vi "Measure.vi"(8 "error in (no error)":errorcluster, 11 "Measurement in":refnum<class "Measurement.lvclass">) -> (0 "error out":errorcluster, 3 "Measurement out":refnum<class "Measurement.lvclass">)   [LabVIEW 2016, in "Measurement Actor.lvlib" / "Measurement.lvclass"]
uses:
  Measurement.lvclass
  C:/Program Files (x86)/National Instruments/LabVIEW 2016/vi.lib/ActorFramework/Actor/Actor.lvclass
  Measurement.lvclass/Measurement.ctl
  <vilib>/ActorFramework/Actor/Actor.lvclass/Actor.ctl
  <vilib>/ActorFramework/Message Enqueuer/Message Enqueuer.lvclass/Message Enqueuer.ctl
  <vilib>/ActorFramework/Message Enqueuer/Init from Existing Queue.vi
  <vilib>/ActorFramework/Message Enqueuer/Enqueue.vi
  Messages/Acquire Msg/Acquire Msg.lvclass
  C:/Program Files (x86)/National Instruments/LabVIEW 2016/vi.lib/ActorFramework/Message/Message.lvclass
  Messages/Close Msg/Close Msg.lvclass
  <vilib>/ActorFramework/Message Priority Queue/Priority Enqueue.vi
  <vilib>/ActorFramework/Message Enqueuer/Message Enqueuer.lvclass
  <vilib>/ActorFramework/Actor/Actor.lvclass
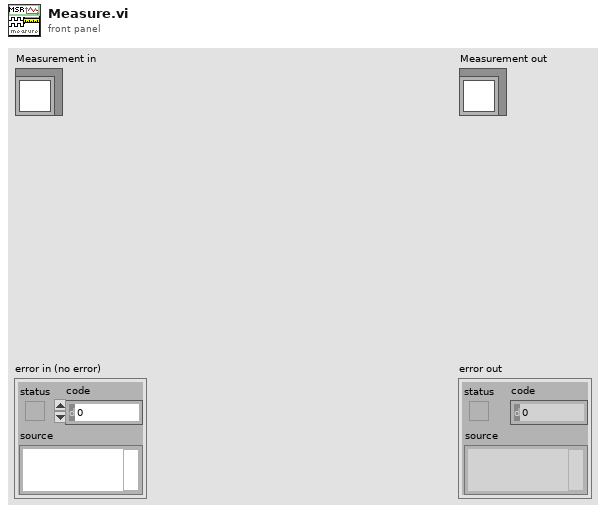
[diagram p1: front panel]
types:
  T1 = typedef "Measurement Actor.lvlib/Measurement.lvclass/Iteration count.ctl" = cluster{"Desired Iterations":i32, "Current":i32}
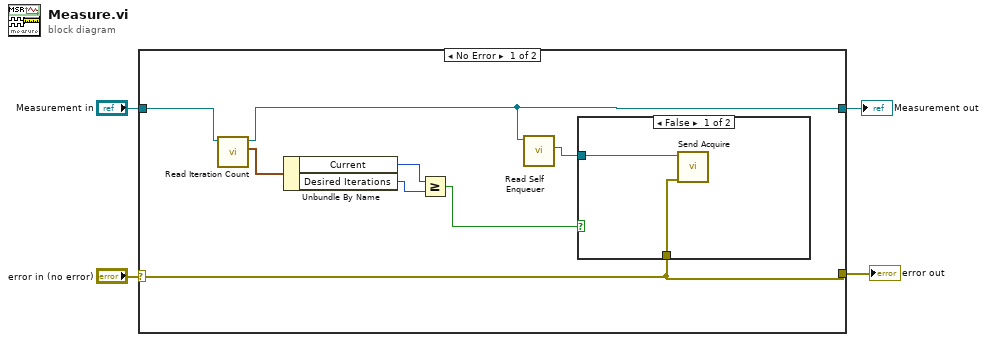
[diagram p0: block diagram]
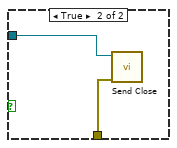
[diagram p2: hidden frame]
diagram:
  n1 = case shown="No Error" "error in (no error)" {
    selector: "error in (no error)" -> [w12 w18]
    tunnel: [w12 w18] -> w3
    tunnel: [w6 w17] -> w1
    tunnel: "Measurement in" -> [w11 w17]
    frame No Error {
      n2 = call "Read Iteration Count.vi"("Measurement in"=w11) -> ("Iteration Count"=w10:T1, "Measurement out"=w6:refnum<class "Measurement.lvclass">)  [unwired: 8 in, 1 out]
      n3 = Unbundle By Name(w10) -> ("Current"=w9:i32, "Desired Iterations"=w8:i32)
      n4 = Greater Or Equal?(x=w9, y=w8) -> (x >= y?=w7:bool)
      n5 = call <vilib>:"Read Self Enqueuer.vi"("Actor"=w6) -> ("Self Enqueuer"=w5:refnum<class "Message Enqueuer.lvclass">)  [unwired: 10 in]
      n6 = case shown="False" w7 {
        tunnel: w12 -> [w13 w16]
        tunnel: w5 -> [w14 w15]
        frame False {
          n7 = call "Send Acquire.vi"("error in (no error)"=w13, "Message Enqueuer in"=w14) -> ()  [unwired: 8 in, 2 out]
        }
        frame True {
          n8 = call "Send Close.vi"("error in (no error)"=w16, "Message Enqueuer in"=w15) -> ()  [unwired: 8 in, 2 out]
        }
      }
    }
    frame Error {
    }
  }
  "error out" <- w3
  "Measurement out" <- w1
